vi "slscsl_initialize.vi"(7 "deviceIdentifier":string, 8 "error in (no error)":errorcluster, 10 "shw file path":path, 11 "Topology in":T1) -> (0 "error out":errorcluster, 3 "slscsl out":refnum<class "slscsl.lvclass">)   [LabVIEW 2017, in "SLSC Switch.lvlib" / "slscsl.lvclass"]
uses:
  slscsl.lvclass
  SLSC Switch/Controls/Topology.ctl
  SLSC Switch/Controls/JSON.InitialState.ctl
  SLSC Switch/Controls/JSON.ChannelList.ctl
  SLSC Switch/Controls/JSON.ConnectionList.ctl
  slscsl.lvclass/slscsl.ctl
  SLSC Switch/SLSC Switch.lvclass
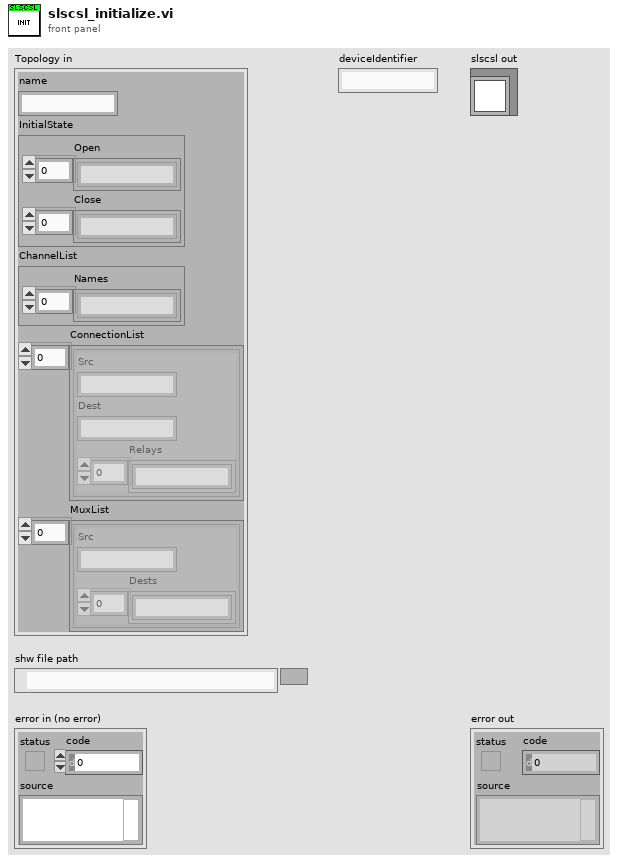
[diagram p1: front panel]
types:
  T1 = typedef "SLSC Switch.lvlib/SLSC Switch.lvclass/Topology.ctl" = cluster{"name":string, "InitialState":T2, "ChannelList":T3, "ConnectionList":T4[], "MuxList":cluster{"Src":string, "Dests":string[]}[]}
  T2 = typedef "SLSC Switch.lvlib/SLSC Switch.lvclass/JSON.InitialState.ctl" = cluster{"Open":string[], "Close":string[]}
  T3 = typedef "SLSC Switch.lvlib/SLSC Switch.lvclass/JSON.ChannelList.ctl" = cluster{"Names":string[]}
  T4 = typedef "SLSC Switch.lvlib/SLSC Switch.lvclass/JSON.ConnectionList.ctl" = cluster{"Src":string, "Dest":string, "Relays":string[]}
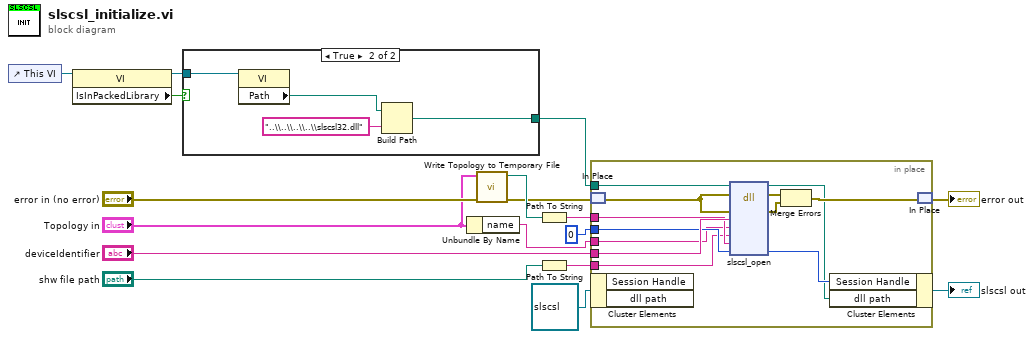
[diagram p0: block diagram]
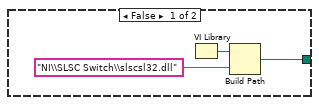
[diagram p2: hidden frame]
diagram:
  n1 = control-ref of="This VI"() -> (w4:refnum<vi>)
  n2 = property class="VI"(reference=w4) -> (reference out=w2:refnum<vi>, "IsInPackedLibrary"=w3:bool)  [unwired: 1 in, 1 out]
  n3 = case shown="True" w3 {
    tunnel: w2 -> [_ w22]
    tunnel: [w18 w23] -> w1
    frame False {
      n4 = VI Library() -> (path=w20:path)
      n5 = Build Path(base path=w20, name or relative path="NI\\SLSC Switch\\slscsl32.dll") -> (appended path=w18:path)
    }
    frame True {
      n6 = property class="VI"(reference=w22) -> ("Path"=w21:path)  [unwired: 1 in, 2 out]
      n7 = Build Path(base path=w21, name or relative path="..\\..\\..\\..\\slscsl32.dll") -> (appended path=w23:path)
    }
  }
  n8 = Unbundle By Name("Topology in") -> ("name"=w5:string)
  n9 = call "Write Topology to Temporary File.vi"("error in (no error)"="error in (no error)", "Topology in"="Topology in") -> ("error out"=w7:errorcluster, "file path"=w9:path)  [unwired: 8 in]
  n10 = Path To String(path=w9) -> (string=w14:string)
  n11 = Path To String(path="shw file path") -> (string=w13:string)
  n12 = in-place {
    in-place-border: "deviceIdentifier" -> [w36]
    in-place-border: u64 0 ("sessionHandlePtr") -> [w35]
    in-place-border: w14 -> [w34]
    in-place-border: w13 -> [w33]
    in-place-border: w5 -> [w27]
    in-place-border: w1 -> [w26]
    n13 = in-place-match #1(w7) -> (w29:errorcluster)
    n14 = in-place-cluster #2(refnum<class "slscsl.lvclass"> refnum ("Route Manager out")) -> ()  [unwired: 2 out]
    n15 = dll-call lib="slscsl*.dll" fn="slscsl_open"(path in=w26, error in=w29, "errorCluster"=w29, "deviceIdentifier"=w36, "topologyName"=w27, "shwFilePath"=w33, "topFilePath"=w34, "sessionHandlePtr"=w35) -> (path out=w25:path, error out=w31:errorcluster, "errorCluster"=w30:errorcluster, "sessionHandlePtr"=w32:u64)  [unwired: 6 in]
    n16 = Merge Errors(w31, w30) -> (w28:errorcluster)
    n17 = in-place-cluster #2("Session Handle"=w32, "dll path"=w25) -> (→"slscsl out":refnum<class "slscsl.lvclass">)
    n18 = in-place-match #1(w28) -> (→"error out":errorcluster)
  }
